vi "MakePath.vi"(1 "Include time":bool, 4 "Index digits":i32=3, 5 "Generate Index":bool=TRUE, 6 "seconds since 1904 (default 0 = now)":u32, 7 "Root Data Folder":path=path "C:/Data", 8 "Error In":errorcluster, 9 "Extentions":string[](array[string])=[".tdms", ".txt", ".tdms_index"], 10 "Interactive":bool=TRUE, 11 "File Prefix":string="s") -> (0 "Error Out":errorcluster, 2 "format string":string="%03d", 3 "Paths out":path[](array[path]))   [LabVIEW 2021]
panel:
  in  "Dashes?":bool
  in  "Split by day":bool=TRUE
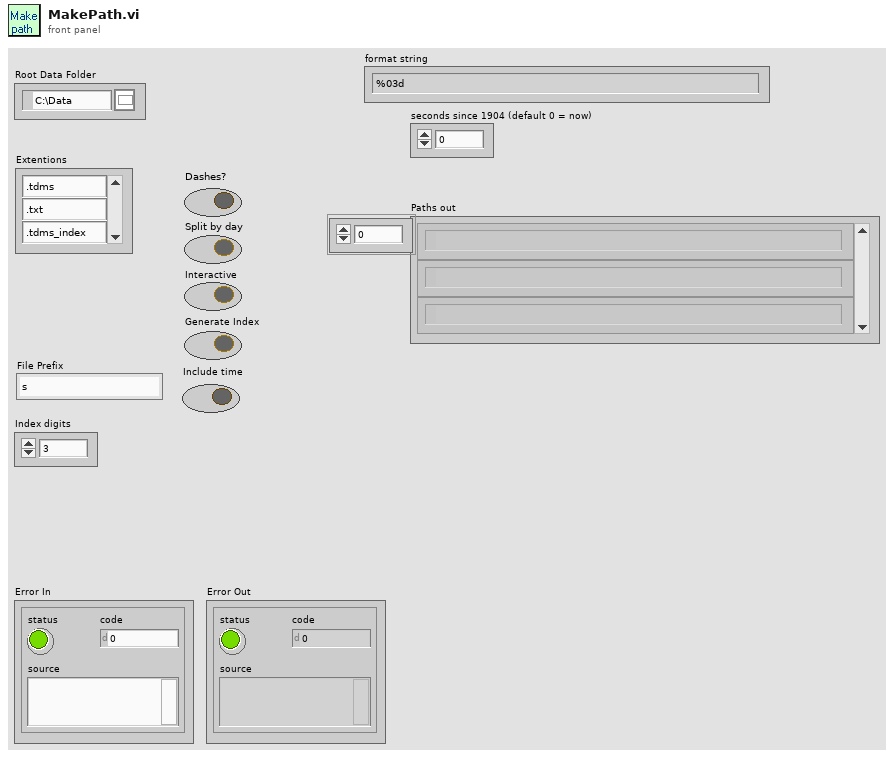
[diagram p1: front panel]
types:
  T1 = enum32{"existing file", "new file", "new or existing file", "existing dir", "new dir", "new or existing dir", "existing file (use LLBs)", "new file (use LLBs)", "new or existing file (use LLBs)", "new or existing file or directory (use LLBs)", "existing dir (use LLBs)", "new dir (use LLBs)", "new or existing dir (use LLBs)", "existing file or dir", "new file or dir", "new or existing file or dir", "existing file or dir (use LLBs)", "new file or dir (use LLBs)"}
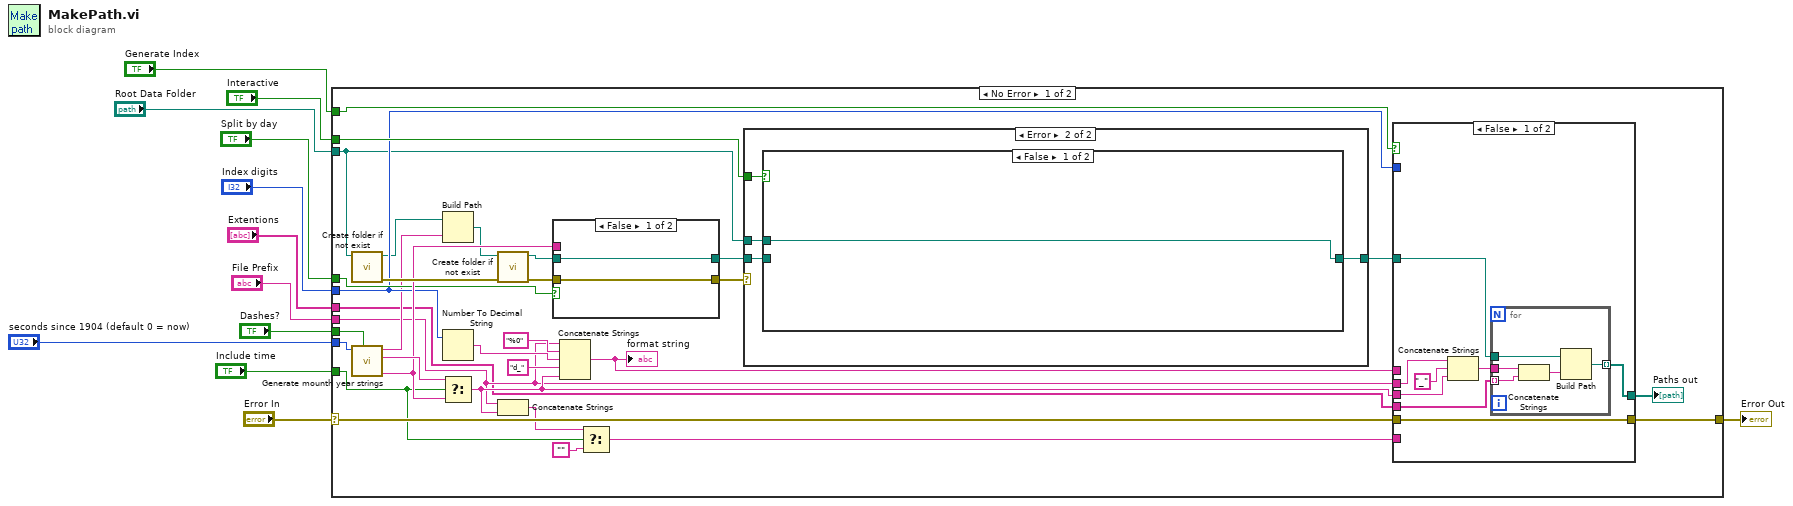
[diagram p0: block diagram]
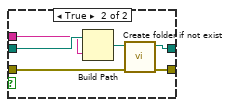
[diagram p2: hidden frame]
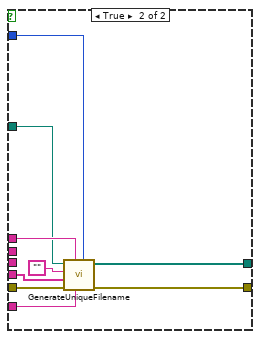
[diagram p3: hidden frame]
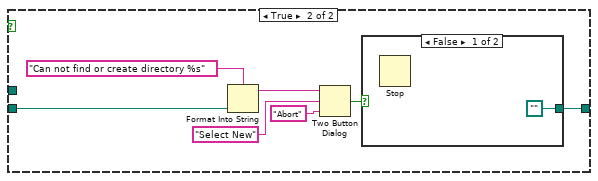
[diagram p5: hidden frame]
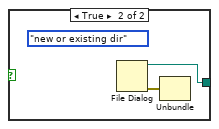
[diagram p6: hidden frame]
diagram:
  n1 = case shown="No Error" "Error In" {
    selector: "Error In" -> [w34 w91]
    tunnel: [w40 w91] -> w11
    tunnel: "Index digits" -> [w19 _]
    tunnel: "seconds since 1904 (default 0 = now)" -> [w25 _]
    tunnel: "Root Data Folder" -> [w15 _]
    tunnel: "Dashes?" -> [w24 _]
    tunnel: "Split by day" -> [w23 _]
    tunnel: "Interactive" -> [w22 _]
    tunnel: "Include time" -> [w21 _]
    tunnel: "Generate Index" -> [w20 _]
    tunnel: "File Prefix" -> [w14 _]
    tunnel: "Extentions" -> [w13 _]
    frame No Error {
      n2 = call "Create folder if not exist.vi"("Folder Path Control"=w15) -> ("Error Out"=w44:errorcluster, "Folder Path out"=w18:path)  [unwired: 1 in, 8 out]
      n3 = call "Generate mounth year strings.vi"("Dashes?"=w24, "seconds since 1904 (default 0 = now)"=w25) -> ("mmdd"=w29:string, "hhmmss_mmdd"=w33:string, "Month_year"=w17:string)  [unwired: 7 out]
      n4 = Build Path(base path=w18, name or relative path=w17) -> (appended path=w16:path)
      n5 = Number To Decimal String(number=w19) -> (decimal integer string=w27:string)  [unwired: 1 in]
      n6 = Select(t=w33, s=w21, f=w29) -> (s? t:f=w28:string)
      n7 = call "Create folder if not exist.vi"("Error In"=w44, "Folder Path Control"=w16) -> ("Error Out"=w42:errorcluster, "Folder Path out"=w43:path)  [unwired: 8 out]
      n8 = Concatenate Strings(w14, w28) -> (w32:string)
      n9 = case shown="False" w23 {
        tunnel: w43 -> [w45 w49]
        tunnel: w42 -> [w46 w52]
        tunnel: [w45 w51] -> w41
        tunnel: [w46 w50] -> w39
        tunnel: w29 -> [_ w48]
        frame False {
        }
        frame True {
          n10 = Build Path(base path=w49, name or relative path=w48) -> (appended path=w47:path)
          n11 = call "Create folder if not exist.vi"("Error In"=w52, "Folder Path Control"=w47) -> ("Error Out"=w50:errorcluster, "Folder Path out"=w51:path)  [unwired: 8 out]
        }
      }
      n12 = Concatenate Strings(w14, "%0" ("Substring"), w27, "d_" ("Substring"), w28) -> (w38:string)
      "format string" <- w38
      n13 = Select(t=w32, s=w21, f="") -> (s? t:f=w31:string)
      n14 = case shown="Error" w39 {
        tunnel: w41 -> [w75 w77]
        tunnel: w22 -> [_ w79]
        tunnel: [w75 w78] -> w36
        tunnel: w15 -> [_ w76]
        frame No Error {
        }
        frame Error {
          n15 = case shown="False" w79 {
            tunnel: [w80 w81] -> w78
            tunnel: w77 -> [_ w85]
            tunnel: w76 -> [w80 _]
            frame False {
            }
            frame True {
              n16 = Format Into String(format string="Can not find or create directory %s" ("Format String"), w85) -> (resulting string=w83:string)  [unwired: 2 in, 1 out]
              n17 = Two Button Dialog(message=w83, 1:"Abort" ("F button name (\"Cancel\")"), 2:"Select New" ("T button name (\"OK\")")) -> (T button?=w82:bool)
              n18 = case shown="False" w82 {
                tunnel: [path "" w90] -> w81
                frame False {
                  n19 = Stop() -> ()  [unwired: 1 out]
                }
                frame True {
                  (unwired) T1."new or existing dir" ("select mode (2)")
                  n20 = File Dialog() -> (0:w89:errorcluster, 3:w90:path)  [unwired: 1 in, 8 out]
                  n21 = Unbundle(w89) -> ()  [unwired: 3 out]
                }
              }
            }
          }
        }
      }
      n22 = case shown="False" w20 {
        tunnel: w28 -> [w58 _]
        tunnel: [w55 w72] -> w35
        tunnel: w36 -> [w53 w66]
        tunnel: w14 -> [w60 _]
        tunnel: [w54 w74] -> w40
        tunnel: w13 -> [w57 w73]
        tunnel: w38 -> [_ w70]
        tunnel: w34 -> [w54 w69]
        tunnel: w31 -> [_ w68]
        tunnel: w19 -> [_ w67]
        frame False {
          n23 = Concatenate Strings(w60, "_" ("Substring"), w58) -> (w56:string)
          n24 = for {
            tunnel: w57 -> [w64] mode=indexing
            tunnel: w56 -> [w65]
            tunnel: [w61] -> w55 mode=indexing
            tunnel: w53 -> [w63]
            n25 = Concatenate Strings(w65, w64) -> (w62:string)
            n26 = Build Path(base path=w63, name or relative path=w62) -> (appended path=w61:path)
          }
        }
        frame True {
          n27 = call "GenerateUniqueFilename.vi"("Index digits"=w67, "No index opion"=w68, "format string"=w70, "Error In"=w69, "File name suffixes"=w73, "File name prefix"="", "Folder Path Control"=w66) -> ("Error Out"=w74:errorcluster, "Paths"=w72:path[])  [unwired: 3 out]
        }
      }
      "Paths out" <- w35
    }
    frame Error {
    }
  }
  "Error Out" <- w11
